vi "HTTP_GET_LV20.vi"(10 "error in (no error)":errorcluster, 11 "Service Link":string) -> (1 "error out":errorcluster, 2 "Reply Body":string, 3 "Reply Header":string)   [LabVIEW 2020]
uses:
  <vilib>/httpClient/LabVIEWHTTPClient.lvlib
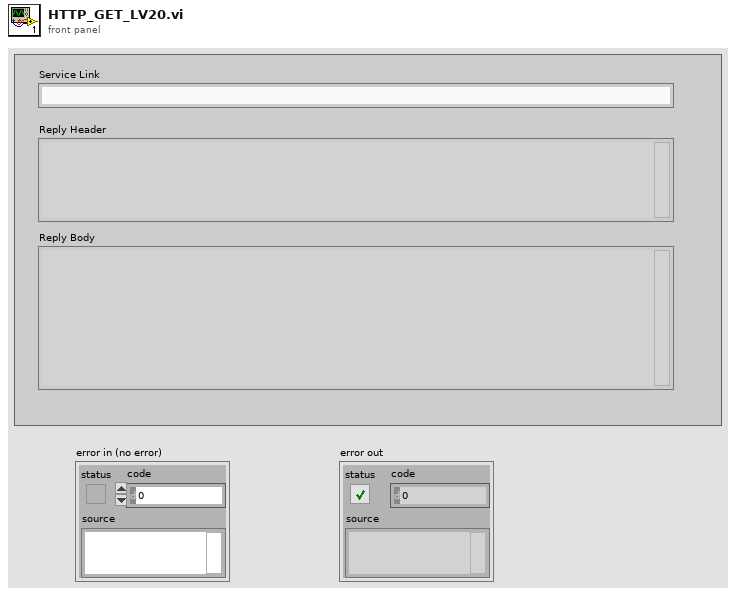
[diagram p1: front panel]
types:
  T1 = typedef "LabVIEWHTTPClient.lvlib/ClientHandle.ctl" = refnum<k1>
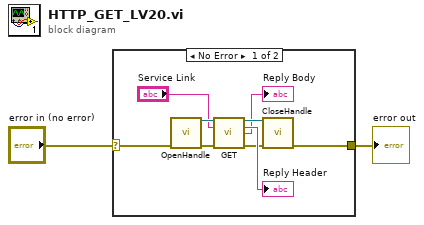
[diagram p0: block diagram]
diagram:
  n1 = case shown="No Error" "error in (no error)" {
    selector: "error in (no error)" -> [w11 w12]
    tunnel: [w10 w12] -> w1
    frame No Error {
      n2 = call <vilib>:"OpenHandle.vi"("error in (no error)"=w11) -> ("client handle out"=w9:T1, "error out"=w7:errorcluster)  [unwired: 13 in]
      n3 = call <vilib>:"GET.vi"("client handle"=w9, "url"="Service Link", "error in (no error)"=w7) -> ("client handle out"=w6:T1, "headers"=→"Reply Header":string, "body"=→"Reply Body":string, "error out"=w3:errorcluster)  [unwired: 9 in]
      n4 = call <vilib>:"CloseHandle.vi"("client handle"=w6, "error in (no error)"=w3) -> ("error out"=w10:errorcluster)  [unwired: 13 in]
    }
    frame Error {
    }
  }
  "error out" <- w1
